vi "WriteMainPanel.vi"(8 "ErrorIn":errorcluster, 10 "MainPanel":refnum<vi>, 11 "ReferenceIn":refnum<class "MasterGUI.lvclass">) -> (0 "ErrorOut":errorcluster, 3 "ReferenceIn":refnum<class "MasterGUI.lvclass">)   [LabVIEW 2021, in "MasterGUI.lvclass"]
uses:
  MasterGUI.lvclass
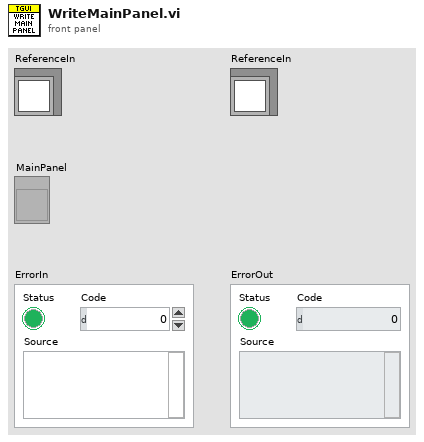
[diagram p1: front panel]
types:
  T1 = typedef "MasterGUI.lvclass/ObjectAttributes.ctl" = cluster{"Interfaces":cluster{"Dummy":refnum<class>}, "Locals":cluster{"MainGUIActive":refnum<queue>, "MainPanel":refnum<vi>, "LayoutPanel":cluster{"PanelVIRef":refnum<vi>, "Labels":string[], "SubPanels":refnum<vi>[]}, "MenuTree":T2[], "Menu":refnum<k9>}, "Persistent":cluster{"StaticDocking":cluster{"ObjectLabel":string, "SubPanelLabel":string}[], "WindowsTitle":string, "AdditionalMenuItems":T2[], "TraceObjectName":string}}
  T2 = typedef "MasterGUI.lvclass/MenuItem.ctl" = cluster{"Parent":string, "Items":string[], "ShortCuts":cluster{"IncludeShiftKey":bool, "IncludeCtrlKey":bool, "ShortcutKey":string}[]}
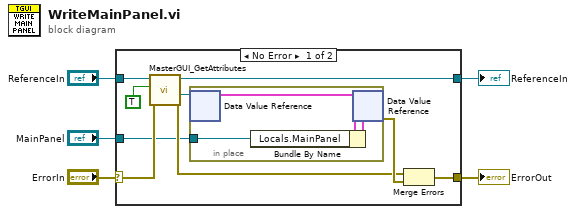
[diagram p0: block diagram]
diagram:
  n1 = case shown="No Error" "ErrorIn" {
    selector: "ErrorIn" -> [w14 w19]
    tunnel: [w11 w19] -> w4
    tunnel: [w9 w18] -> w2
    tunnel: "ReferenceIn" -> [w10 w18]
    tunnel: "MainPanel" -> [w6 _]
    frame No Error {
      n2 = call "MasterGUI_GetAttributes.vi"("ErrorIn"=w14, "OnlyGetDvrReference(False)"=TRUE, "ReferenceIn"=w10) -> ("ErrorOut"=w12:errorcluster, "DataRef"=w7:refnum<data-value>, "ReferenceOut"=w9:refnum<class "MasterGUI.lvclass">)  [unwired: 5 in, 1 out]
      n3 = in-place {
        in-place-border: w6 -> [w15]
        n4 = in-place-dvr #1(w7) -> (w16:T1)  [unwired: 1 out]
        n5 = Bundle By Name(cluster=w16, "Locals.MainPanel"=w15) -> (w17:T1)
        n6 = in-place-dvr #1(w17) -> (w13:errorcluster)  [unwired: 1 out]
      }
      n7 = Merge Errors(w12, w13) -> (w11:errorcluster)
    }
    frame Error {
    }
  }
  "ErrorOut" <- w4
  "ReferenceIn" <- w2
